vi "Main.vi"() -> ()   [LabVIEW 2019]
doc: "This template is for the Queued Message Handler design pattern.\n\nThe Event Handling Loop generates messages based on user interface actions.\n\nThe Message Handling Loop processes messages generated by the Event Handling Loop, or by other messages. The messages are string values, so new messages can be added easily to the Message Cases case structure in the Message Handling Loop. Each message cluster can also provide an optional value for Message Data, which is a variant that can be converted to whatever message-specific data is required."
uses:
  controls/UI Data.ctl
  support/Message Queue/Enqueue Message (Single).vi
  <vilib>/Utility/error.llb/Error Cluster From Error Code.vi
  support/Message Queue/Enqueue Message (Array).vi
  <vilib>/ErrorRing/Error Ring.xnode
  support/Message Queue/Message Queue.lvlib
  support/User Event - Stop/User Event - Stop.lvlib
panel:
  in  "Error en MHL":bool
  in  "Error en EHL":bool
  out "Meter":dbl(knob) scale=0.0..10.0
  in  "Knob":dbl(knob) scale=0.0..10.0
  out "Display <Replace Me>":string
  in  "Do Something Else <Replace Me>":bool
  in  "Do Something <Replace Me>":bool
  in  "Exit":bool
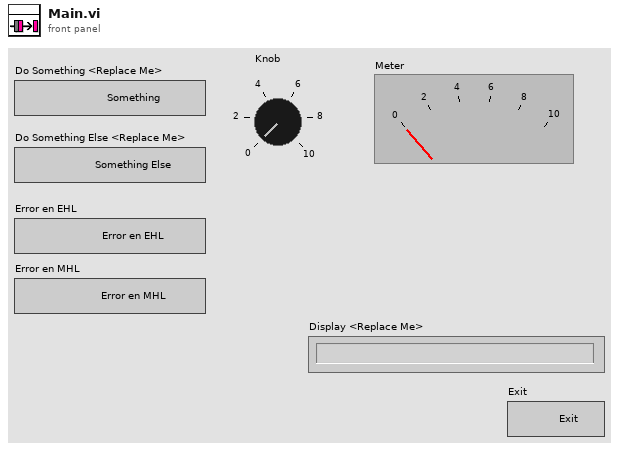
[diagram p1: front panel]
types:
  T1 = typedef "UI Data.ctl" = cluster{"Boolean <Replace Me>":bool, "String <Replace Me>":string, "Numeric <Replace Me>":dbl, "Do Something Ref":refnum<vi>, "Do Something Else Ref":refnum<vi>, "Data Display Ref":refnum<vi>, "Exit Button Ref":refnum<vi>}
  T2 = typedef "Message Queue.lvlib/All Message Queues.ctl" = cluster{"UI":refnum<queue>}
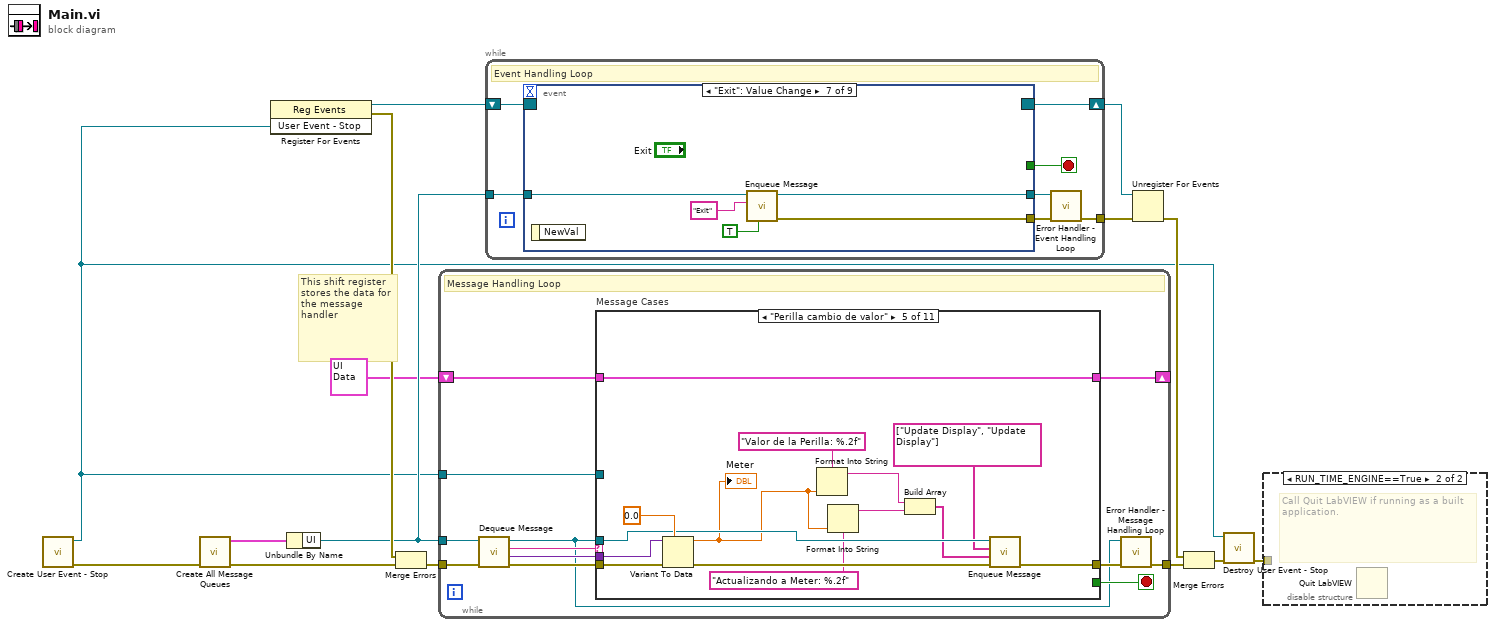
[diagram p0: block diagram]
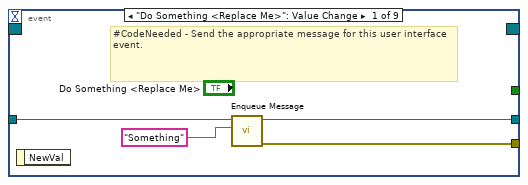
[diagram p3: hidden frame]
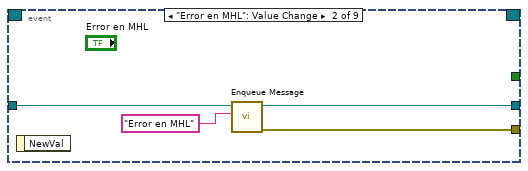
[diagram p4: hidden frame]
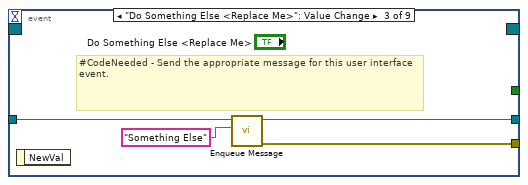
[diagram p5: hidden frame]
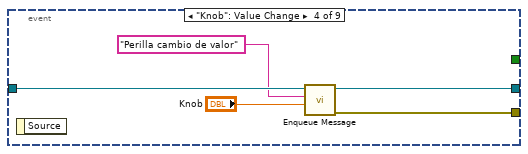
[diagram p6: hidden frame]
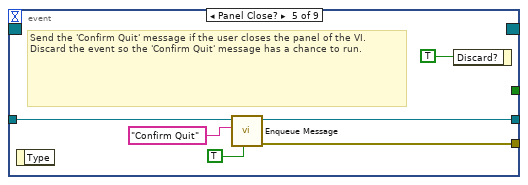
[diagram p7: hidden frame]
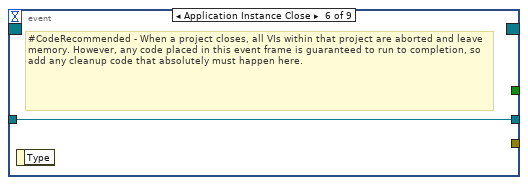
[diagram p8: hidden frame]
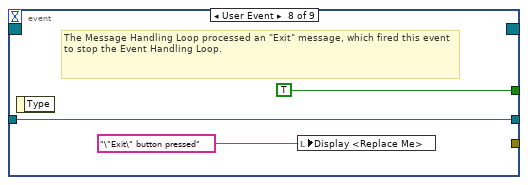
[diagram p9: hidden frame]
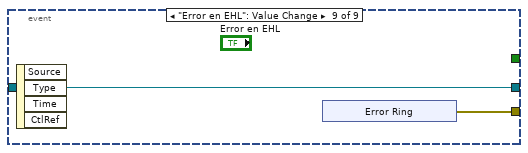
[diagram p10: hidden frame]
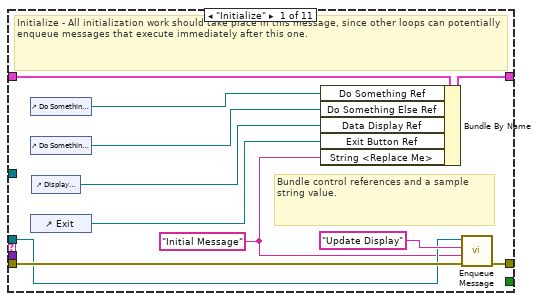
[diagram p11: hidden frame]
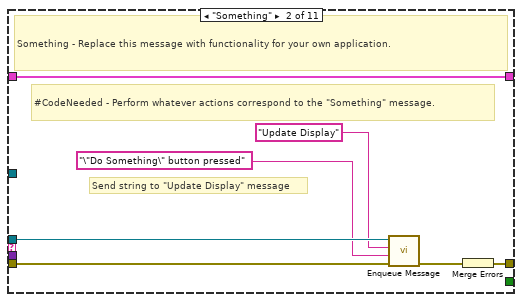
[diagram p12: hidden frame]
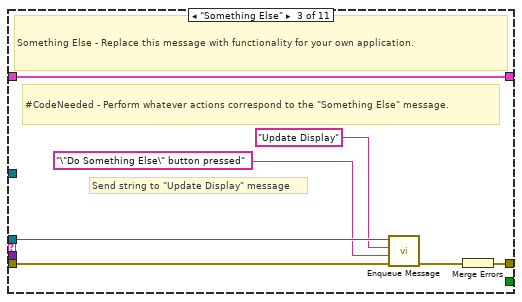
[diagram p13: hidden frame]
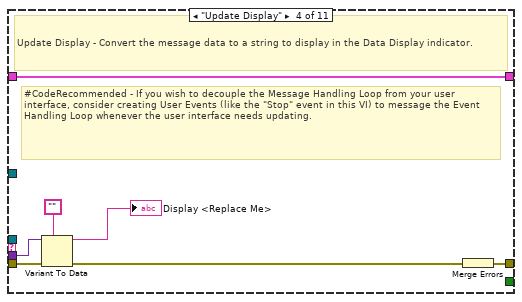
[diagram p14: hidden frame]
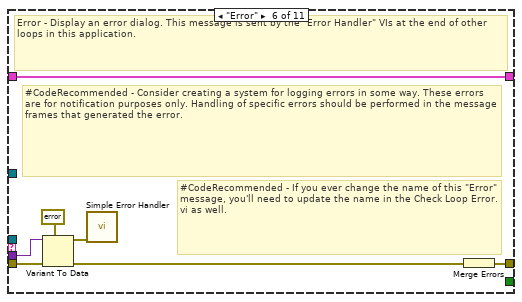
[diagram p15: hidden frame]
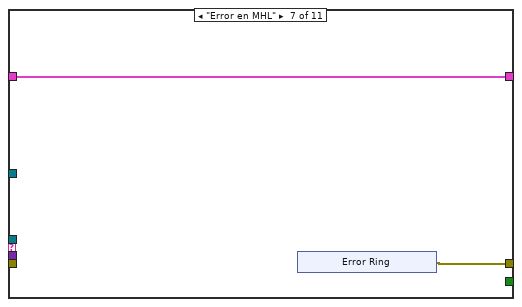
[diagram p16: hidden frame]
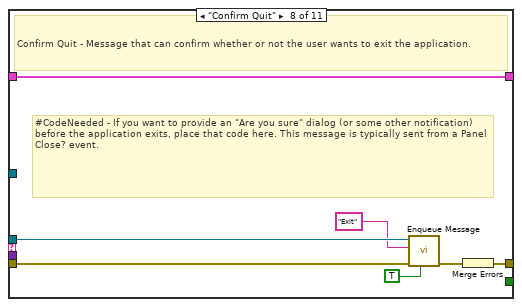
[diagram p17: hidden frame]
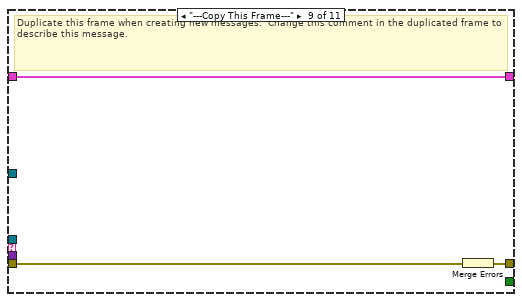
[diagram p18: hidden frame]
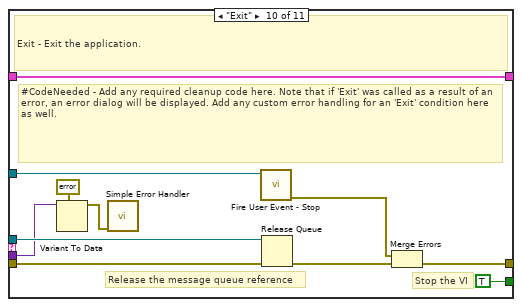
[diagram p19: hidden frame]
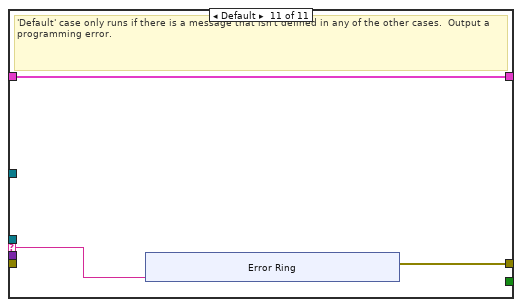
[diagram p20: hidden frame]
diagram:
  # "This shift register stores the data for the message handler"
  n1 = call "Create User Event - Stop.vi"() -> ("error out"=w13:errorcluster, "User Event - Stop"=w1:refnum<user-event>)  [unwired: 10 in]
  n2 = call "Create All Message Queues.vi"("error in (no error)"=w13) -> ("error out"=w15:errorcluster, "Message Queues out"=w6:T2)  [unwired: 9 in]
  n3 = register-events(w1) -> (reference out=w2:refnum<event-registration>, error out=w7:errorcluster)  [unwired: 2 in]
  n4 = Unbundle By Name(w6) -> ("UI"=w5:refnum<queue>)
  n5 = Merge Errors(w7, w15) -> (w8:errorcluster)
  n6 = while {
    tunnel: w5 -> [w17]
    shift-right: [w22] -> _
    shift-left: T1 {"Boolean <Replace Me>"=FALSE, "String <Replace Me>"="", "Numeric <Replace Me>"=0.0, "Do Something Ref"=refnum, "Do Something Else Ref"=refnum, "Data Display Ref"=refnum, "Exit Button Ref"=refnum} ("Data Cluster") -> [w23]
    tunnel: w1 -> [w20]
    tunnel: w8 -> [w27]
    tunnel: [w25] -> w14
    stop <- w21 stop-if-true
    # "Message Handling Loop"
    n7 = call "Dequeue Message.vi"("error in (no error)"=w27, "Message Queue"=w17) -> ("error out"=w26:errorcluster, "Message Data"=w18:variant, "Message"=w19:string, "dup Message Queue"=w16:refnum<queue>)  [unwired: 6 in]
    n8 = case "Message Cases" shown="\"Perilla cambio de valor\"" w19 {
      selector: w19 -> [_ _ _ _ _ _ _ _ _ _ w109]
      tunnel: w16 -> [w29 w41 w48 _ w67 _ _ w90 _ w102 _]
      tunnel: w26 -> [w37 w44 w51 w58 w73 w80 _ w94 w97 w105 _]
      tunnel: [w38 w45 w52 w59 w68 w76 w81 w93 w96 w107 w111] -> w24
      tunnel: w23 -> [w36 w42 w49 w56 w72 w75 w82 w91 w95 w101 w110]
      tunnel: [w35 w42 w49 w56 w72 w75 w82 w91 w95 w101 w110] -> w22
      tunnel: [_ _ _ _ _ _ _ _ _ TRUE _] -> w21
      tunnel: w18 -> [_ _ _ w55 w70 w74 _ _ _ w98 _]
      tunnel: w20 -> [_ _ _ _ _ _ _ _ _ w99 _]
      frame "Initialize" {
        w28 = "Initial Message" ("Initial Message")
        # "Bundle control references and a sample string value."
        # "Initialize - All initialization work should take place in this message, since other loops can potentially enqueue messages that execute immediately after this one."
        n9 = control-ref of="Do Something <Replace Me>"() -> (w34:refnum<vi>)
        n10 = control-ref of="Do Something Else <Replace Me>"() -> (w33:refnum<vi>)
        n11 = control-ref of="Exit"() -> (w31:refnum<vi>)
        n12 = control-ref of="Display <Replace Me>"() -> (w32:refnum<vi>)
        n13 = Bundle By Name(cluster=w36, "Do Something Ref"=w34, "Do Something Else Ref"=w33, "Data Display Ref"=w32, "Exit Button Ref"=w31, "String <Replace Me>"=w28) -> (w35:T1)
        n14 = call-poly "Enqueue Message.vi"("error in (no error)"=w37, "Message Data"=w28, "Message"="Update Display", "Message Queue"=w29) -> ("error out"=w38:errorcluster)  [unwired: 6 in, 1 out]
      }
      frame "Something" {
        # "Send string to \"Update Display\" message"
        # "#CodeNeeded - Perform whatever actions correspond to the \"Something\" message."
        # "Something - Replace this message with functionality for your own application."
        n15 = call-poly "Enqueue Message.vi"("error in (no error)"=w44, "Message Data"="\"Do Something\" button pressed" ("\"Do Something\" button pressed"), "Message"="Update Display", "Message Queue"=w41) -> ("error out"=w43:errorcluster)  [unwired: 6 in, 1 out]
        n16 = Merge Errors(w43) -> (w45:errorcluster)
      }
      frame "Something Else" {
        # "Send string to \"Update Display\" message"
        # "#CodeNeeded - Perform whatever actions correspond to the \"Something Else\" message."
        # "Something Else - Replace this message with functionality for your own application."
        n17 = call-poly "Enqueue Message.vi"("error in (no error)"=w51, "Message Data"="\"Do Something Else\" button pressed" ("\"Do Something Else\" button pressed"), "Message"="Update Display", "Message Queue"=w48) -> ("error out"=w50:errorcluster)  [unwired: 6 in, 1 out]
        n18 = Merge Errors(w50) -> (w52:errorcluster)
      }
      frame "Update Display" {
        # "#CodeRecommended - If you wish to decouple the Message Handling Loop from your user interface, consider creating User Events (like the \"Stop\" event in this VI) to message the Event Handling Loop whenever the user interface needs updating."
        # "Update Display - Convert the message data to a string to display in the Data Display indicator."
        n19 = Variant To Data(error in=w58, type="", Variant=w55) -> (data=→"Display <Replace Me>":string, error out=w57:errorcluster)
        n20 = Merge Errors(w57) -> (w59:errorcluster)
      }
      frame "Perilla cambio de valor" {
        n21 = Variant To Data(error in=w73, type=0.0, Variant=w70) -> (data=w64:dbl, error out=w71:errorcluster)
        "Meter" <- w64
        n22 = Format Into String(format string="Valor de la Perilla: %.2f", w64) -> (resulting string=w61:string)  [unwired: 2 in, 1 out]
        n23 = Format Into String(format string="Actualizando a Meter: %.2f", w64) -> (resulting string=w62:string)  [unwired: 2 in, 1 out]
        n24 = Build Array(w61, w62) -> (w60:string[])
        n25 = call-poly "Enqueue Message.vi"("error in (no error)"=w71, "Message Data Array"=w60, "Message Array"=string[] ["Update Display", "Update Display"] ("Message"), "Message Queue"=w67) -> ("error out"=w68:errorcluster)  [unwired: 6 in, 1 out]
      }
      frame "Error" {
        # "#CodeRecommended - If you ever change the name of this \"Error\" message, you'll need to update the name in the Check Loop Error.vi as well."
        # "#CodeRecommended - Consider creating a system for logging errors in some way. These errors are for notification purposes only. Handling of specific errors should be performed in the message frames that generated the error."
        # "Error - Display an error dialog. This message is sent by the \"Error Handler\" VIs at the end of other loops in this application."
        n26 = Variant To Data(error in=w80, type=errorcluster {"status"=FALSE, "code"=0, "source"=""} ("error constant"), Variant=w74) -> (data=w78:errorcluster, error out=w77:errorcluster)
        n27 = call <vilib>:"Simple Error Handler.vi"("error in (no error)"=w78) -> ()  [unwired: 4 in, 5 out]
        n28 = Merge Errors(w77) -> (w76:errorcluster)
      }
      frame "Error en MHL" {
        n29 = xnode "Error Ring"() -> ("error out"=w81:errorcluster)
      }
      frame "Confirm Quit" {
        # "#CodeNeeded - If you want to provide an \"Are you sure\" dialog (or some other notification) before the application exits, place that code here. This message is typically sent from a Panel Close? event."
        # "Confirm Quit - Message that can confirm whether or not the user wants to exit the application."
        n30 = call-poly "Enqueue Message.vi"("Priority Message? (F)"=TRUE, "error in (no error)"=w94, "Message"="Exit", "Message Queue"=w90) -> ("error out"=w92:errorcluster)  [unwired: 6 in, 1 out]
        n31 = Merge Errors(w92) -> (w93:errorcluster)
      }
      frame "---Copy This Frame---" {
        # "Duplicate this frame when creating new messages.  Change this comment in the duplicated frame to describe this message."
        n32 = Merge Errors(w97) -> (w96:errorcluster)
      }
      frame "Exit" {
        # "Stop the VI"
        # "Release the message queue reference"
        # "#CodeNeeded - Add any required cleanup code here. Note that if 'Exit' was called as a result of an error, an error dialog will be displayed. Add any custom error handling for an 'Exit' condition here as well."
        # "Exit - Exit the application."
        n33 = Variant To Data(type=errorcluster {"status"=FALSE, "code"=0, "source"=""} ("error constant"), Variant=w98) -> (data=w103:errorcluster)  [unwired: 1 in, 1 out]
        n34 = call <vilib>:"Simple Error Handler.vi"("error in (no error)"=w103) -> ()  [unwired: 4 in, 5 out]
        n35 = call "Fire User Event - Stop.vi"("User Event - Stop"=w99) -> ("error out"=w106:errorcluster)  [unwired: 10 in]
        n36 = Release Queue(queue=w102, error in (no error)=w105) -> (error out=w108:errorcluster)  [unwired: 1 in, 2 out]
        n37 = Merge Errors(w106, w108) -> (w107:errorcluster)
      }
      frame Default {
        # "'Default' case only runs if there is a message that isn't defined in any of the other cases.  Output a programming error."
        n38 = xnode "Error Ring"("parameter 0"=w109) -> ("error out"=w111:errorcluster)
      }
    }
    n39 = call "Error Handler - Message Handling Loop.vi"("error in (no error)"=w24, "Message Queue"=w16) -> ("dup error in"=w25:errorcluster)  [unwired: 8 in, 1 out]
  }
  n40 = while {
    tunnel: w5 -> [w123]
    shift-right: [w121] -> w4
    shift-left: w2 -> [w122]
    tunnel: [w124] -> w9
    stop <- w120 stop-if-true
    # "Event Handling Loop"
    n41 = event shown="[6] \"Exit\": Value Change" {
      selector: w122 -> [_ _ _ _ _ _ _ _ _]
      dyn-events: [_ _ _ _ _ _ _ _ _] -> w121
      timeout: _ -> [_ _ _ _ _ _ _ _ _]
      tunnel: [_ _ _ _ _ _ _ TRUE ("Discard?") _] -> w120
      tunnel: w123 -> [w128 w132 w136 w142 w146 w149 w153 w157 w159]
      tunnel: [w129 w133 w137 w138 w148 _ w154 _ w158] -> w125
      tunnel: [w127 w131 w135 w141 w145 w149 w152 w157 w159] -> w119
      event "Do Something <Replace Me>": Value Change {
        # "#CodeNeeded - Send the appropriate message for this user interface event."
        n42 = event-data() -> ()  [unwired: 1 in, 1 out]
        n43 = call-poly "Enqueue Message.vi"("Message"="Something", "Message Queue"=w128) -> ("error out"=w129:errorcluster, "dup Message Queue"=w127:refnum<queue>)  [unwired: 8 in]
      }
      event "Error en MHL": Value Change {
        n44 = event-data() -> ()  [unwired: 1 in, 1 out]
        n45 = call-poly "Enqueue Message.vi"("Message"="Error en MHL", "Message Queue"=w132) -> ("error out"=w133:errorcluster, "dup Message Queue"=w131:refnum<queue>)  [unwired: 8 in]
      }
      event "Do Something Else <Replace Me>": Value Change {
        # "#CodeNeeded - Send the appropriate message for this user interface event."
        n46 = event-data() -> ()  [unwired: 1 in, 1 out]
        n47 = call-poly "Enqueue Message.vi"("Message"="Something Else", "Message Queue"=w136) -> ("error out"=w137:errorcluster, "dup Message Queue"=w135:refnum<queue>)  [unwired: 8 in]
      }
      event "Knob": Value Change {
        n48 = event-data() -> ()  [unwired: 1 in, 1 out]
        n49 = call-poly "Enqueue Message.vi"("Message Data"="Knob", "Message"="Perilla cambio de valor", "Message Queue"=w142) -> ("error out"=w138:errorcluster, "dup Message Queue"=w141:refnum<queue>)  [unwired: 7 in]
      }
      event Panel Close? {
        # "Send the 'Confirm Quit' message if the user closes the panel of the VI. Discard the event so the 'Confirm Quit' message has a chance to run."
        n50 = event-data() -> ()  [unwired: 1 in, 1 out]
        n51 = call-poly "Enqueue Message.vi"("Priority Message? (F)"=TRUE, "Message"="Confirm Quit", "Message Queue"=w146) -> ("error out"=w148:errorcluster, "dup Message Queue"=w145:refnum<queue>)  [unwired: 7 in]
        n52 = event-data("Discard?"=TRUE) -> ()  [unwired: 1 in, 1 out]
      }
      event Application Instance Close {
        # "#CodeRecommended - When a project closes, all VIs within that project are aborted and leave memory. However, any code placed in this event frame is guaranteed to run to completion, so add any cleanup code that absolutely must happen here."
        n53 = event-data() -> ()  [unwired: 1 in, 1 out]
      }
      event "Exit": Value Change {
        n54 = event-data() -> ()  [unwired: 1 in, 1 out]
        n55 = call-poly "Enqueue Message.vi"("Priority Message? (F)"=TRUE, "Message"="Exit", "Message Queue"=w153) -> ("error out"=w154:errorcluster, "dup Message Queue"=w152:refnum<queue>)  [unwired: 7 in]
      }
      event User Event {
        # "The Message Handling Loop processed an \"Exit\" message, which fired this event to stop the Event Handling Loop."
        n56 = event-data() -> ()  [unwired: 1 in, 1 out]
        n57 = local write "Display <Replace Me>"("\"Exit\" button pressed" ("VI Stopped")) -> ()
      }
      event "Error en EHL": Value Change {
        n58 = event-data() -> ()  [unwired: 1 in, 4 out]
        n59 = xnode "Error Ring"() -> ("error out"=w158:errorcluster)
      }
    }
    n60 = call "Error Handler - Event Handling Loop.vi"("error in (no error)"=w125, "Message Queue"=w119) -> ("dup error in"=w124:errorcluster)  [unwired: 8 in, 1 out]
  }
  n61 = Unregister For Events(event registration refnum=w4, error in=w9) -> (error out=w11:errorcluster)
  n62 = Merge Errors(w11, w14) -> (w12:errorcluster)
  n63 = call "Destroy User Event - Stop.vi"("error in (no error)"=w12, "User Event - Stop"=w1) -> ("error out"=w10:errorcluster)  [unwired: 9 in]
  n64 = disable-structure shown="RUN_TIME_ENGINE==True" {
    disable-tunnel: w10 -> [_ _]
    frame condition #0 (active) {
    }
    frame condition #1 {
      # "Call Quit LabVIEW if running as a built application."
      n65 = Quit LabVIEW() -> ()  [unwired: 1 in]
    }
  }
